vi "Num Ref Get U32 String.vi"(8 "error in (no error)":errorcluster, 11 "U32 Ref":refnum<vi>) -> (0 "error out":errorcluster, 3 "Value string":string)   [LabVIEW 2018, in "Main Panel.lvlib" / "Main Panel.lvclass"]
uses:
  Main Panel.lvclass
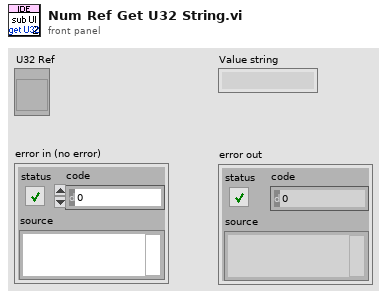
[diagram p1: front panel]
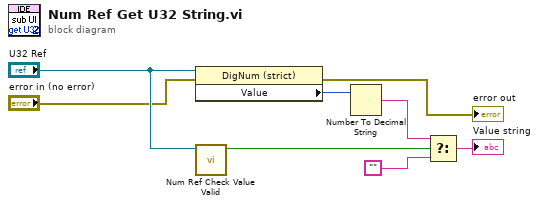
[diagram p0: block diagram]
diagram:
  n1 = property class="DigNum (strict)"(reference="U32 Ref", error in="error in (no error)") -> (error out=→"error out":errorcluster, "Value"=w8:u32)  [unwired: 1 out]
  n2 = call "Num Ref Check Value Valid.vi"("Num Ref"="U32 Ref") -> ("Valid"=w5:bool)  [unwired: 9 in, 1 out]
  n3 = Number To Decimal String(number=w8) -> (decimal integer string=w4:string)  [unwired: 1 in]
  n4 = Select(t=w4, s=w5, f="") -> (s? t:f=→"Value string":string)
